vi "PLC-WriteValues.vi"(8 "error in":errorcluster, 10 "Slot":i32, 11 "Idx":i32) -> (0 "error out":errorcluster)   [LabVIEW 2016]
doc: "Go to PLC->SaveToDB action\n\nWabco 2017 All right reserved\nAuthor: maciej.szupienko@wabco-auto.com"
uses:
  PLC.Action.ctl
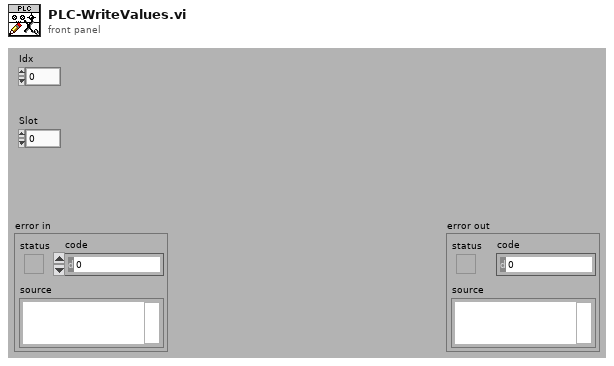
[diagram p1: front panel]
types:
  T1 = typedef "PLC.Action.ctl" = enum32{"idle", "constructor", "destructor", "-- PLC --", "Setup", "WriteValues", "GetPrevStatus", "GetProdComp", "AddProdComp"}
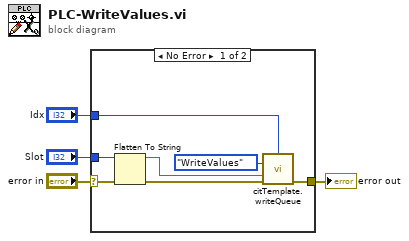
[diagram p0: block diagram]
diagram:
  n1 = case shown="No Error" "error in" {
    selector: "error in" -> [w11 w12]
    tunnel: [w10 w12] -> w3
    tunnel: "Idx" -> [w8 _]
    tunnel: "Slot" -> [w6 _]
    frame No Error {
      n2 = Flatten To String(anything=w6, error in (no error)=w11) -> (data string=w5:string, error out=w7:errorcluster)  [unwired: 2 in, 1 out]
      n3 = call "citTemplate.writeQueue.vi"("instance (0)"=w8, "event in (if not connected:all statemachine with data event)"=PLC.Action."WriteValues" ("Action"), "data in"=w5, "error in (no error)"=w7) -> ("error out"=w10:errorcluster)  [unwired: 11 in]
    }
    frame Error {
    }
  }
  "error out" <- w3
